vi "Create.vi"(8 "error in (no error)":errorcluster) -> (0 "error out":errorcluster, 3 "Identical Inputs Comparator":refnum<class "Identical Arguments Comparator.lvclass">)   [LabVIEW 2020, in "Identical Arguments Comparator.lvclass"]
uses:
  Identical Arguments Comparator.lvclass
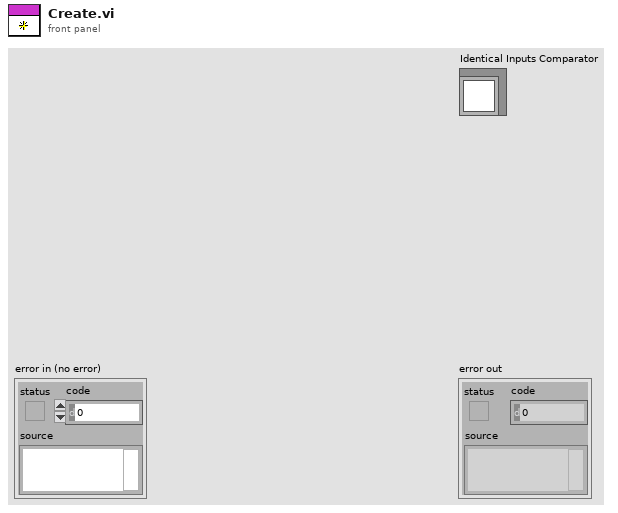
[diagram p1: front panel]
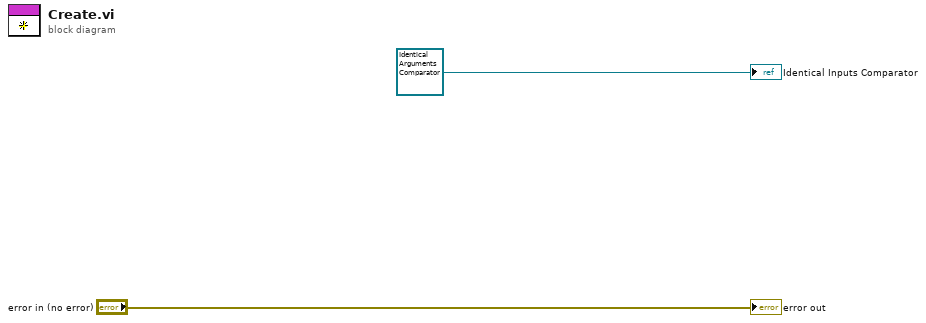
[diagram p0: block diagram]
diagram:
  "error out" <- "error in (no error)"
  "Identical Inputs Comparator" <- refnum<class "Identical Arguments Comparator.lvclass"> refnum ("Identical Inputs Comparator")
